vi "e.gate Decode UDBF.vi"   [LabVIEW 2016]
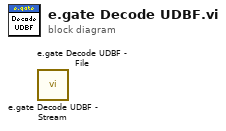
[diagram p0: block diagram]
diagram:
  n1 = call "e.gate Decode UDBF - Stream.vi"() -> ()  [unwired: 9 in, 3 out]
  n2 = call "e.gate Decode UDBF - File.vi"() -> ()  [unwired: 9 in, 3 out]
